vi "CloseSensorSession.vi"(8 "error in (no error)":errorcluster, 11 "SiemensDigitalEnergyMeter in":refnum<class "SiemensDigitalEnergyMeter.lvclass">) -> (0 "error out":errorcluster, 3 "SiemensDigitalEnergyMeter out":refnum<class "SiemensDigitalEnergyMeter.lvclass">)   [LabVIEW 2018, in "SensorPlugins.lvlib" / "SiemensDigitalEnergyMeter.lvclass"]
doc: "This VI closes the communicaiton link to the Siemens Digital Energy Meter from the application."
uses:
  SiemensDigitalEnergyMeter.lvclass
  <vilib>/NI/Modbus Library/API/Master/Modbus Master.lvclass
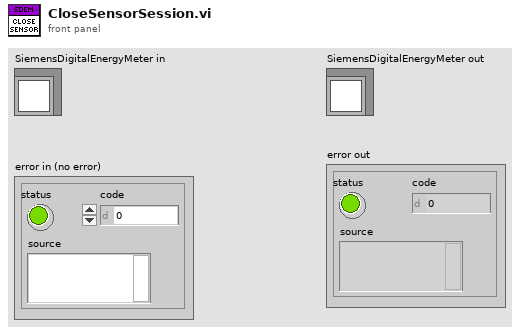
[diagram p1: front panel]
types:
  T1 = typedef "SensorPlugins.lvlib/SiemensDigitalEnergyMeter.lvclass/SiemensDigitalEnergyMeterControls.ctl" = cluster{"Measurement(s)":u16[], "Configuration Commands":string, "Use Measurement Commands Text Box?":bool, "Measurement Commands":string, "Connected?":bool, "Serial Number":string, "IP Address":string, "Port (502)":u16, "Unit ID":u8, "Serial Type":enum16{"RTU", "ASCII"}, "Using TCP?":bool, "VISA Resource Name":string}[]
  T2 = typedef "SensorPlugins.lvlib/SiemensDigitalEnergyMeter.lvclass/CommunicationControls.ctl" = refnum<class "Modbus Master.lvclass">[]
  T3 = cluster{"Measurement(s)":u16[], "Configuration Commands":string, "Use Measurement Commands Text Box?":bool, "Measurement Commands":string, "Connected?":bool, "Serial Number":string, "IP Address":string, "Port (502)":u16, "Unit ID":u8, "Serial Type":enum16{"RTU", "ASCII"}, "Using TCP?":bool, "VISA Resource Name":string}
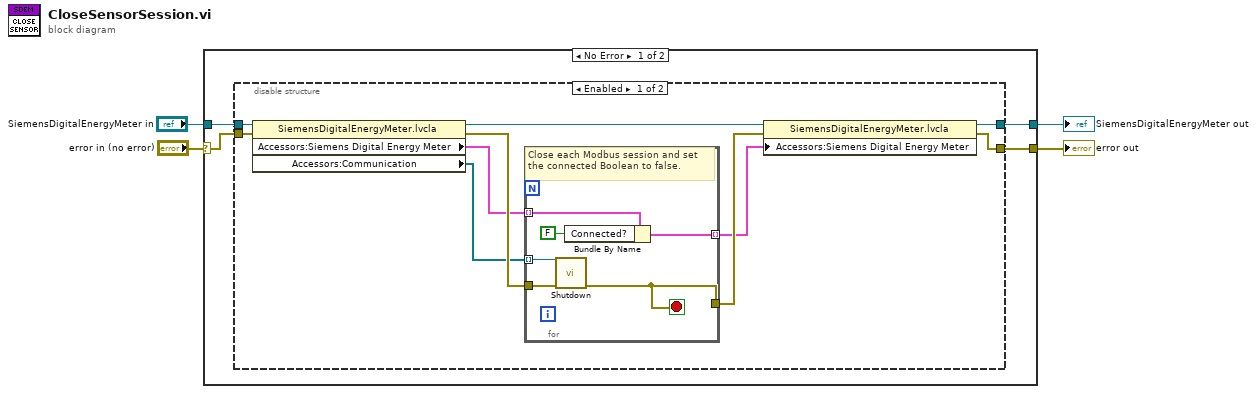
[diagram p0: block diagram]
diagram:
  n1 = case shown="No Error" "error in (no error)" {
    selector: "error in (no error)" -> [w7 w27]
    tunnel: "SiemensDigitalEnergyMeter in" -> [w8 w28]
    tunnel: [w6 w28] -> w2
    tunnel: [w5 w27] -> w1
    frame No Error {
      n2 = disable-structure shown="Enabled" {
        disable-tunnel: w8 -> [w18 w26]
        disable-tunnel: w7 -> [w17 w25]
        disable-tunnel: [w14 w26] -> w6
        disable-tunnel: [w13 w25] -> w5
        frame Enabled {
          n3 = property class="SiemensDigitalEnergyMeter.lvcla"(reference=w18, error in=w17) -> (reference out=w15:refnum<class "SiemensDigitalEnergyMeter.lvclass">, error out=w16:errorcluster, "Accessors:Siemens Digital Energy Meter"=w10:T1, "Accessors:Communication"=w9:T2)
          n4 = for {
            tunnel: w16 -> [w24]
            tunnel: [w23] -> w12
            tunnel: w9 -> [w22] mode=indexing
            tunnel: w10 -> [w21] mode=indexing
            tunnel: [w19] -> w11 mode=indexing
            stop <- w23 stop-if-true
            # "Close each Modbus session and set the connected Boolean to false."
            n5 = call-dynamic "Shutdown.vi"("error in"=w24, "Modbus master in"=w22) -> ("error out"=w23:errorcluster)  [unwired: 9 in]
            n6 = Bundle By Name(cluster=w21, "Connected?"=FALSE) -> (w19:T3)
          }
          n7 = property class="SiemensDigitalEnergyMeter.lvcla"(reference=w15, error in=w12, "Accessors:Siemens Digital Energy Meter"=w11) -> (reference out=w14:refnum<class "SiemensDigitalEnergyMeter.lvclass">, error out=w13:errorcluster)
        }
        frame Disabled {
        }
      }
    }
    frame Error {
    }
  }
  "error out" <- w1
  "SiemensDigitalEnergyMeter out" <- w2
